vi "LEP_RV_CompilerFlags.vi"(1 "Generate Integer Only":bool, 2 "Show compile warnings":bool, 3 "Build configuration":u16(ring) items=["Debug", "Release"]) -> (0 "CFlags":string)   [LabVIEW 2011]
doc: "Returns the compiler flags to use when building an embedded VI into an embedded application."
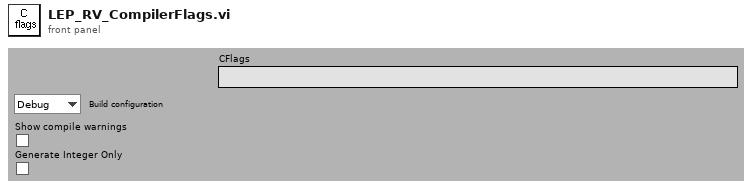
[diagram p1: front panel]
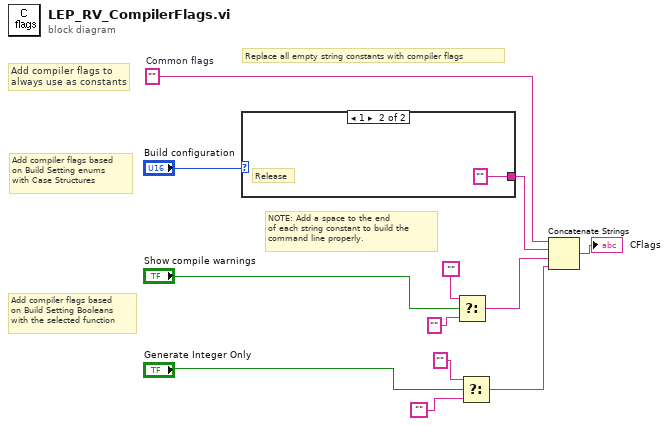
[diagram p0: block diagram]
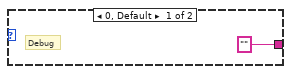
[diagram p2: hidden frame]
diagram:
  w2 = ""  # Common flags
  # "Replace all empty string constants with compiler flags"
  # "NOTE: Add a space to the end\nof each string constant to build the\ncommand line properly."
  # "Add compiler flags based\non Build Setting Booleans\nwith the selected function"
  # "Add compiler flags based\non Build Setting enums\nwith Case Structures"
  # "Add compiler flags to\nalways use as constants"
  n1 = case shown="1" "Build configuration" {
    tunnel: ["" ""] -> w1
    frame 0, Default {
      # "Debug"
    }
    frame 1 {
      # "Release"
    }
  }
  n2 = Select(t="", s="Show compile warnings", f="") -> (s? t:f=w7:string)
  n3 = Select(t="", s="Generate Integer Only", f="") -> (s? t:f=w6:string)
  n4 = Concatenate Strings(w2, w1, w7, w6) -> (→"CFlags":string)
